vi "process_error_handler.vi"() -> ()   [LabVIEW 2011, in "Fiberscope_library.lvlib"]
uses:
  Fiberscope_library.lvlib
  typedefs/main_state_cluster.ctl
  typedefs/main_state_enum.ctl
  globals/global_exit.vi
panel:
  out "Error?":T1
  out "error out":errorcluster
  in  "error in (no error)":errorcluster
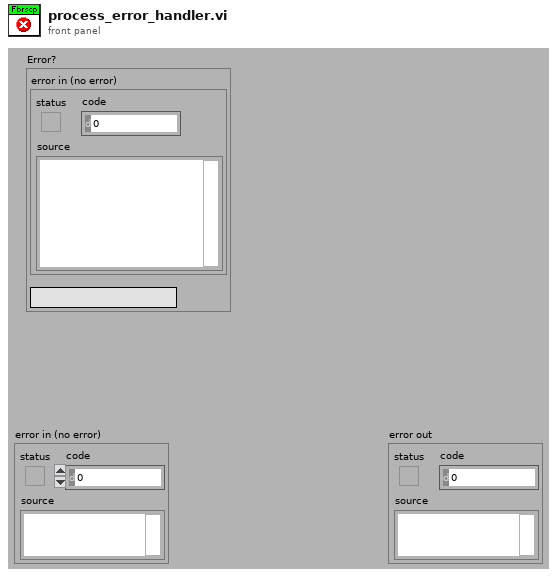
[diagram p1: front panel]
types:
  T1 = cluster{"error in (no error)":errorcluster, string}
  T2 = typedef "Fiberscope_library.lvlib/main_state_cluster.ctl" = cluster{"Main_state_enum":T3, "State_data_variant":variant}
  T3 = typedef "Fiberscope_library.lvlib/main_state_enum.ctl" = enum16{"Init", "Error", "Quit", "Run", "Stop", "Change_parameters", "Timeout", "Shutter", "Save", "Wait_for_finished", "Change_storage", "Change_pixelmap", "Change_averages", "Run_finished", "Change_runmode"}
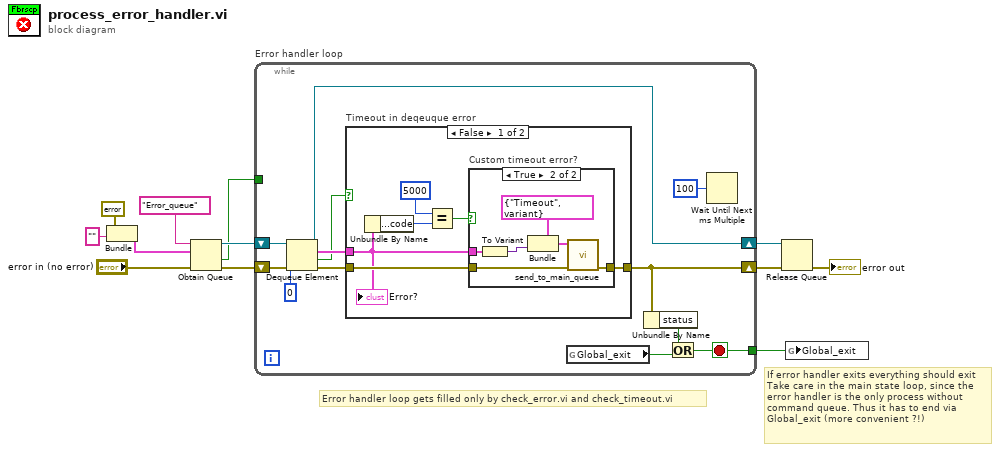
[diagram p0: block diagram]
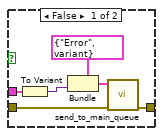
[diagram p2: hidden frame]
diagram:
  # "Error handler loop gets filled only by check_error.vi and check_timeout.vi"
  # "If error handler exits everything should exit\nTake care in the main state loop, since the\nerror handler is the only process without\ncommand queue. Thus it has to end via\nGlobal_exit (more convenient ?!)"
  n1 = Bundle("error in (no error)"=errorcluster {"status"=FALSE, "code"=0, "source"=""}, "") -> (w1:T1)  [unwired: 1 in]
  n2 = Obtain Queue(name (unnamed)="Error_queue", element data type=w1, error in (no error)="error in (no error)") -> (queue out=w9:refnum<queue>, created new?=w4:bool, error out=w10:errorcluster)  [unwired: 2 in]
  n3 = while "Error handler loop" {
    shift-right: [w20] -> w8
    shift-left: w10 -> [w24]
    tunnel: [w18] -> w5
    shift-right: [w21] -> w7
    shift-left: w9 -> [w23]
    tunnel: w4 -> [_]
    stop <- w18 stop-if-true
    n4 = Dequeue Element(queue=w23, timeout in ms (-1)=0, error in (no error)=w24) -> (queue out=w21:refnum<queue>, element=w22:T1, timed out?=w14:bool, error out=w13:errorcluster)
    n5 = case "Timeout in deqeuque error" shown="False" w14 {
      tunnel: w22 -> [w25 _]
      tunnel: [w30 w43] -> w20
      tunnel: w13 -> [w29 w43]
      frame False {
        n6 = Unbundle By Name(w25) -> ("error in (no error).code"=w28:i32)
        n7 = Equal?(x=5000, y=w28) -> (x = y?=w26:bool)
        n8 = case "Custom timeout error?" shown="True" w26 {
          tunnel: [w36 w42] -> w30
          tunnel: w29 -> [w35 w41]
          tunnel: w25 -> [w34 w40]
          frame False {
            n9 = To Variant(anything=w34) -> (Variant=w32:variant)
            n10 = Bundle(cluster=T2 {"Main_state_enum"=enum."Error", "State_data_variant"=variant} ("Main_state_cluster"), "State_data_variant"=w32) -> (w33:T2)  [unwired: 1 in]
            n11 = call "send_to_main_queue.vi"("error in (no error)"=w35, "Main_state_cluster"=w33) -> ("error out"=w36:errorcluster)  [unwired: 9 in]
          }
          frame True {
            n12 = To Variant(anything=w40) -> (Variant=w38:variant)
            n13 = Bundle(cluster=T2 {"Main_state_enum"=enum."Timeout", "State_data_variant"=variant} ("Main_state_cluster"), "State_data_variant"=w38) -> (w39:T2)  [unwired: 1 in]
            n14 = call "send_to_main_queue.vi"("error in (no error)"=w41, "Main_state_cluster"=w39) -> ("error out"=w42:errorcluster)  [unwired: 9 in]
          }
        }
        "Error?" <- w25
      }
      frame True {
      }
    }
    n15 = global read "global_exit.vi" "Global_exit"() -> (w16:bool)
    n16 = Unbundle By Name(w20) -> ("status"=w19:bool)
    n17 = Or(x=w19, y=w16) -> (x .or. y?=w18:bool)
    n18 = Wait Until Next ms Multiple(millisecond multiple=u32 100) -> ()  [unwired: 1 out]
  }
  n19 = Release Queue(queue=w7, error in (no error)=w8) -> (error out=→"error out":errorcluster)  [unwired: 1 in, 2 out]
  n20 = global write "global_exit.vi" "Global_exit"(w5) -> ()
